vi "RMS value.vi"() -> ()   [LabVIEW 2018]
uses:
  <vilib>/Analysis/5stat.llb/RMS (DBL).vi
  <vilib>/Analysis/NI_AALPro.lvlib
panel:
  out "RMS":dbl
  in  "String":string
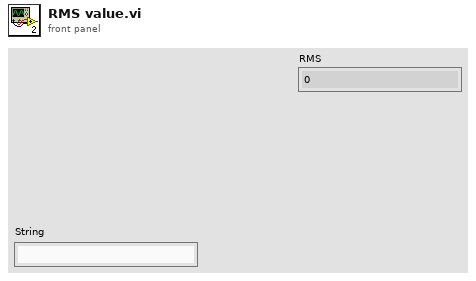
[diagram p1: front panel]
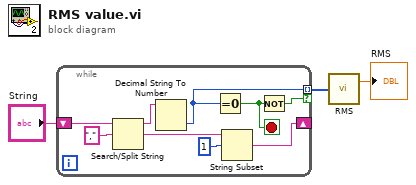
[diagram p0: block diagram]
diagram:
  n1 = while {
    shift-right: [w8] -> _
    shift-left: "String" -> [w9]
    tunnel: [w6] -> w2 mode=indexing if=w4
    stop <- w5 stop-if-true
    n2 = Search/Split String(string=w9, search string/char (-)=",") -> (substring before match=w7:string, match + rest of string=w11:string)  [unwired: 1 in, 1 out]
    n3 = Decimal String To Number(string=w7) -> (number=w6:i32)  [unwired: 2 in, 1 out]
    n4 = Equal To 0?(x=w6) -> (x = 0?=w5:bool)
    n5 = String Subset(string=w11, offset (0)=1) -> (substring=w8:string)  [unwired: 1 in]
    n6 = Not(x=w5) -> (.not. x?=w4:bool)
  }
  n7 = call-poly <vilib>:"RMS.vi"("X"=w2) -> ("rms value"=→"RMS":dbl)  [unwired: 1 out]
